vi "custom vi connector template.vi"(9 "customQueue":refnum<queue>, 11 "parentQueue":refnum<queue>) -> ()   [LabVIEW 2018]
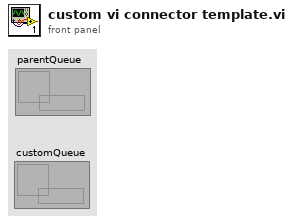
[diagram p1: front panel]
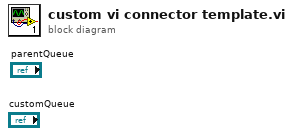
[diagram p0: block diagram]
diagram:
